vi "CSM Check - State.vi"(8 "Matched Previous?":bool, 10 "Cross CSM Data (In)":T1={"Name (\"\" to Use UUID)"="", "Current State"="", "Arguments"="", "Source Message"={"‘State"="", "’Arguments"="", "’Error"={"status"=FALSE, "code"=0, "source"=""}}, "Source Module"="", "Complete(T)/Start(F)"=FALSE, "LogType"=enum."State Change", "Time Stamp"=timestamp(0 s since 1904-01-01)}, 11 "GlobalLogFilter.lvclass":refnum<class "LogFilter.lvclass">) -> (0 "Matched? (Dup)":bool, 2 "Cross CSM Data":T1={"Name (\"\" to Use UUID)"="", "Current State"="", "Arguments"="", "Source Message"={"‘State"="", "’Arguments"="", "’Error"={"status"=FALSE, "code"=0, "source"=""}}, "Source Module"="", "Complete(T)/Start(F)"=FALSE, "LogType"=enum."State Change", "Time Stamp"=timestamp(0 s since 1904-01-01)}, 3 "GlobalLogFilter.lvclass (Dup)":refnum<class "LogFilter.lvclass">)   [LabVIEW 2017, in "Communicable State Machine.lvlib" / "LogFilter.lvclass"]
doc: "### CSM Check - State.vi\n\n-- <b>Controls</b> --\n- <b>Matched Previous?</b>:\n- <b>Cross CSM Data (in)</b>:\n- <b>GlobalLogFilter.lvclass</b>:\n\n-- <b>Indicators</b> --\n- <b>Matched? (dup)</b>:\n- <b>Cross CSM Data</b>:\n- <b>GlobalLogFilter.lvclass (dup)</b>:"
uses:
  LogFilter.lvclass
  Typedef/_CSM_GlobalLog_MSG.ctl
  Typedef/_CSM_Response Source Message.ctl
  Typedef/_CSM_GlobalLog_MSG_TYPE.ctl
  LogFilter.lvclass/LogFilter.ctl
  Communicable State Machine.lvlib
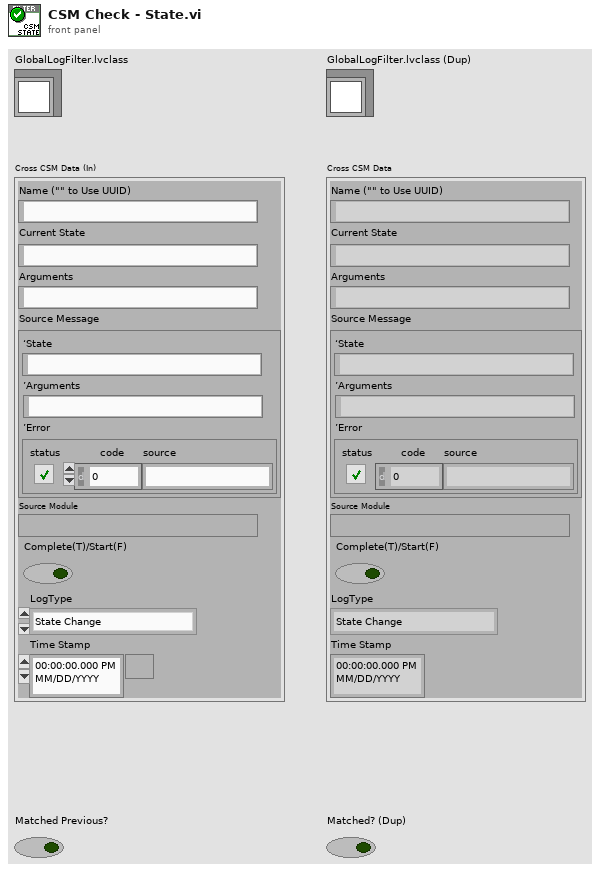
[diagram p1: front panel]
types:
  T1 = typedef "Communicable State Machine.lvlib/_CSM_GlobalLog_MSG.ctl" = cluster{"Name (\"\" to Use UUID)":string, "Current State":string, "Arguments":string, "Source Message":T2, "Source Module":string, "Complete(T)/Start(F)":bool, "LogType":T3, "Time Stamp":timestamp}
  T2 = typedef "Communicable State Machine.lvlib/_CSM_Response Source Message.ctl" = cluster{"‘State":string, "’Arguments":string, "’Error":errorcluster}
  T3 = typedef "Communicable State Machine.lvlib/_CSM_GlobalLog_MSG_TYPE.ctl" = enum16{"User Log", "State Change", "Status", "Interrupt", "Register", "Unregister", "Error Log", "Module Created", "Module Destroyed", "Async Message", "No-Rep Async Message", "Sync Message", "AsyncMsg Complete", "SyncMsg Complete"}
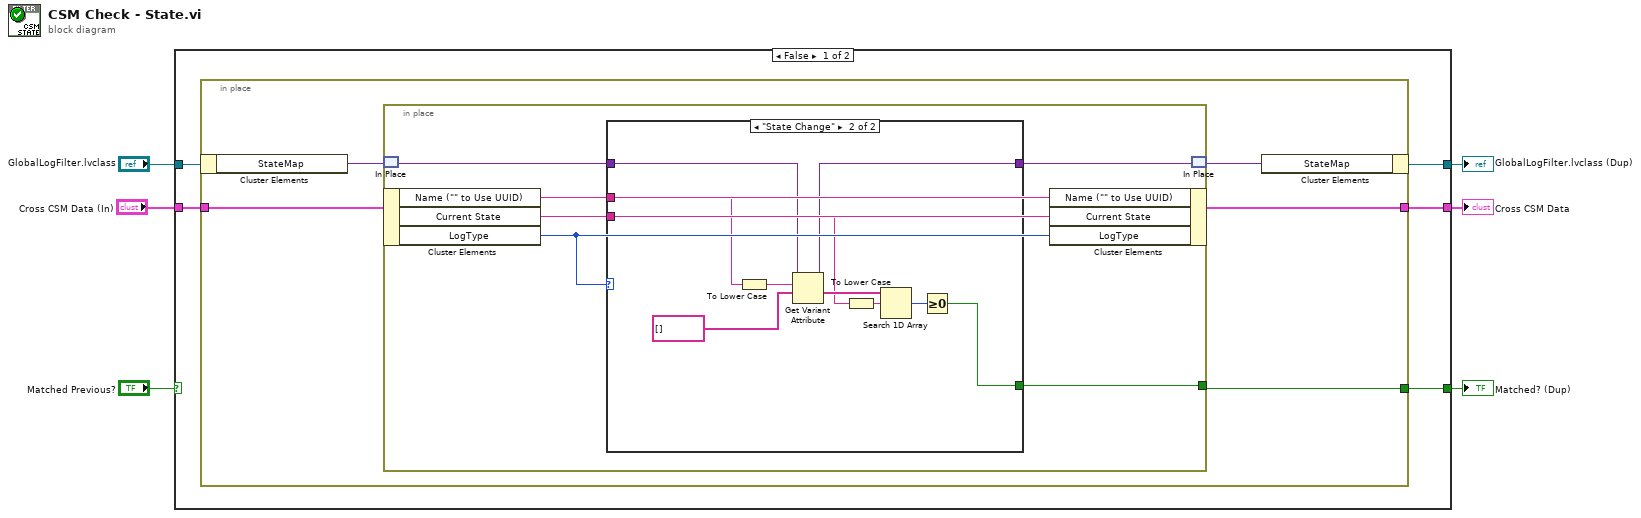
[diagram p0: block diagram]
diagram:
  n1 = case shown="False" "Matched Previous?" {
    selector: "Matched Previous?" -> [_ w35]
    tunnel: [w10 w36] -> w5
    tunnel: "Cross CSM Data (In)" -> [w11 w36]
    tunnel: [w9 w35] -> w3
    tunnel: [w7 w34] -> w2
    tunnel: "GlobalLogFilter.lvclass" -> [w8 w34]
    frame False {
      n2 = in-place {
        in-place-border: w11 -> [w16]
        in-place-border: [w15] -> w10
        in-place-border: [w14] -> w9
        n3 = in-place-cluster #1(w8) -> ("StateMap"=w13:variant)
        n4 = in-place {
          in-place-border: [w18] -> w14
          n5 = in-place-match #2(w13) -> (w22:variant)
          n6 = in-place-cluster #3(w16) -> ("Name (\"\" to Use UUID)"=w20:string, "Current State"=w19:string, "LogType"=w17:T3)
          n7 = case shown="\"State Change\"" w17 {
            tunnel: w22 -> [w23 w33]
            tunnel: [w23 w32] -> w21
            tunnel: w20 -> [_ w31]
            tunnel: w19 -> [_ w28]
            tunnel: [_ w26] -> w18
            frame Default {
            }
            frame "State Change" {
              n8 = To Lower Case(string=w31) -> (all lower case string=w25:string)
              n9 = Get Variant Attribute(Variant=w33, name=w25, default value (empty Variant)=string[] []) -> (duplicate Variant=w32:variant, value=w29:string[])  [unwired: 1 in, 2 out]
              n10 = To Lower Case(string=w28) -> (all lower case string=w24:string)
              n11 = Search 1D Array(1D array=w29, element=w24) -> (index of element=w27:i32)  [unwired: 1 in]
              n12 = Greater Or Equal To 0?(x=w27) -> (x >= 0?=w26:bool)
            }
          }
          n13 = in-place-cluster #3("Name (\"\" to Use UUID)"=w20, "Current State"=w19, "LogType"=w17) -> (w15:T1)
          n14 = in-place-match #2(w21) -> (w12:variant)
        }
        n15 = in-place-cluster #1("StateMap"=w12) -> (w7:refnum<class "LogFilter.lvclass">)
      }
    }
    frame True {
    }
  }
  "Cross CSM Data" <- w5
  "Matched? (Dup)" <- w3
  "GlobalLogFilter.lvclass (Dup)" <- w2
